vi "array of vectors -- algebra.vi"(4 "Array in":dbl[](array[numeric])=[0.1, 0.25, 0.5, 0.75, 1.25, 1.5], 6 "number":dbl=1.0, 7 "?":T2=enum."random", 8 "vec IN":cluster{"center x":dbl, "center Y":dbl}, 9 "Matrix":T1, 10 "y IN":dbl[](array[numeric])=[0.0, 0.0, 0.0, 0.0, 0.0, 0.0, 0.0, 0.0, 0.0, 0.0, 0.0, 0.0, 0.0, 0.0, 0.0, 0.0, 0.0, 0.0, 0.0, 0.0], 11 "x IN":dbl[](array[numeric])=[0.0, 0.0, 0.0, 0.0, 0.0, 0.0, 0.0, 0.0, 0.0, 0.0, 0.0, 0.0, 0.0, 0.0, 0.0, 0.0, 0.0, 0.0, 0.0, 0.0]) -> (0 "z out":dbl[](array[numeric]), 2 "y IOUT":dbl[](array[numeric])=[-0.10773170361060114, 0.457772952697413, -0.009555100977947983, -0.48804447463777656, -0.09984232901729184, 0.13119560893774174, -0.22283442709873946, 0.3059520406815761, -0.2724761090008474, 0.4459726318517574, 0.374683420003999, 0.15733456556750114, -0.2681733941926512, -0.18835513867488007, 0.201519355363871, -0.42899488425478816, 0.017153200329568463, -0.07357806321342775, -0.03965505008312653, -0.24040362888086708, 0.034052108855892715, 0.31924689447313703, -0.10598568269389563, -0.4403683770100004, -0.39067866845839583, -0.07628563470535954, 0.4798388214319522, 0.11632430011978867, 0.028320122257029068, -0.3713197715201815, 0.3687635262719211, -0.1672236935026572, -0.17019816064120863, 0.2670856862236137, -0.018456225948212834, -0.3697432881980798, 0.45329130138320917, 0.291174819494997, -0.4775794640153177, 0.20278732148372658, 0.00010603725885349746, -0.2782732301335482, -0.3370559874481738, -0.03489202794563595, 0.0441236466978302, 0.014425835304824552, 0.25050858523876185, 0.04621463682703997, 0.3475519129062037, 0.20029679806376333], 3 "x  OUT":dbl[](array[numeric])=[0.40090360765964794, 0.40170449063806646, 0.3719833615168324, -0.41942074860305834, 0.23408694456181145, 0.2004301402449875, -0.27413414162219407, 0.3227096166685155, -0.13636471969040254, -0.3615712316380595, -0.30837390549735244, -0.4972725670503759, 0.4538715795393323, -0.28219588600377743, -0.015344431033755601, -0.03162125419338757, 0.10462141481001197, -0.2184998697199254, -0.22600023642322253, -0.4336430625371366, -0.35474597926419627, -0.17008105009388963, 0.11680613183230104, -0.3147381858650824, 0.01810260701745814, 0.08118463453483504, 0.13197188439702667, -0.21774239766248127, -0.11943352032855747, 0.2300723285374393, 0.2763664885251238, -0.007778949200884622, 0.43387299574285265, 0.4591137756966033, 0.2612719864618036, -0.012468509690670038, -0.45450783010510687, -0.016721282298933993, -0.2893390780903706, 0.06254002811272952, 0.40529670225894754, -0.18315282359791607, 0.24745070704533223, 0.19736719755441556, -0.06565361009683168, 0.3076490949601618, -0.027569391016634803, -0.41363424870437493, 0.028513782340929383, 0.3932763712837244])   [LabVIEW 2021]
uses:
  array of vectors -- algebra.ctl
  <vilib>/Analysis/Matrix/Datatypes/RealMatrix.ctl
  generate linear region.vi
  <vilib>/Analysis/Matrix/NI_Matrix.lvlib
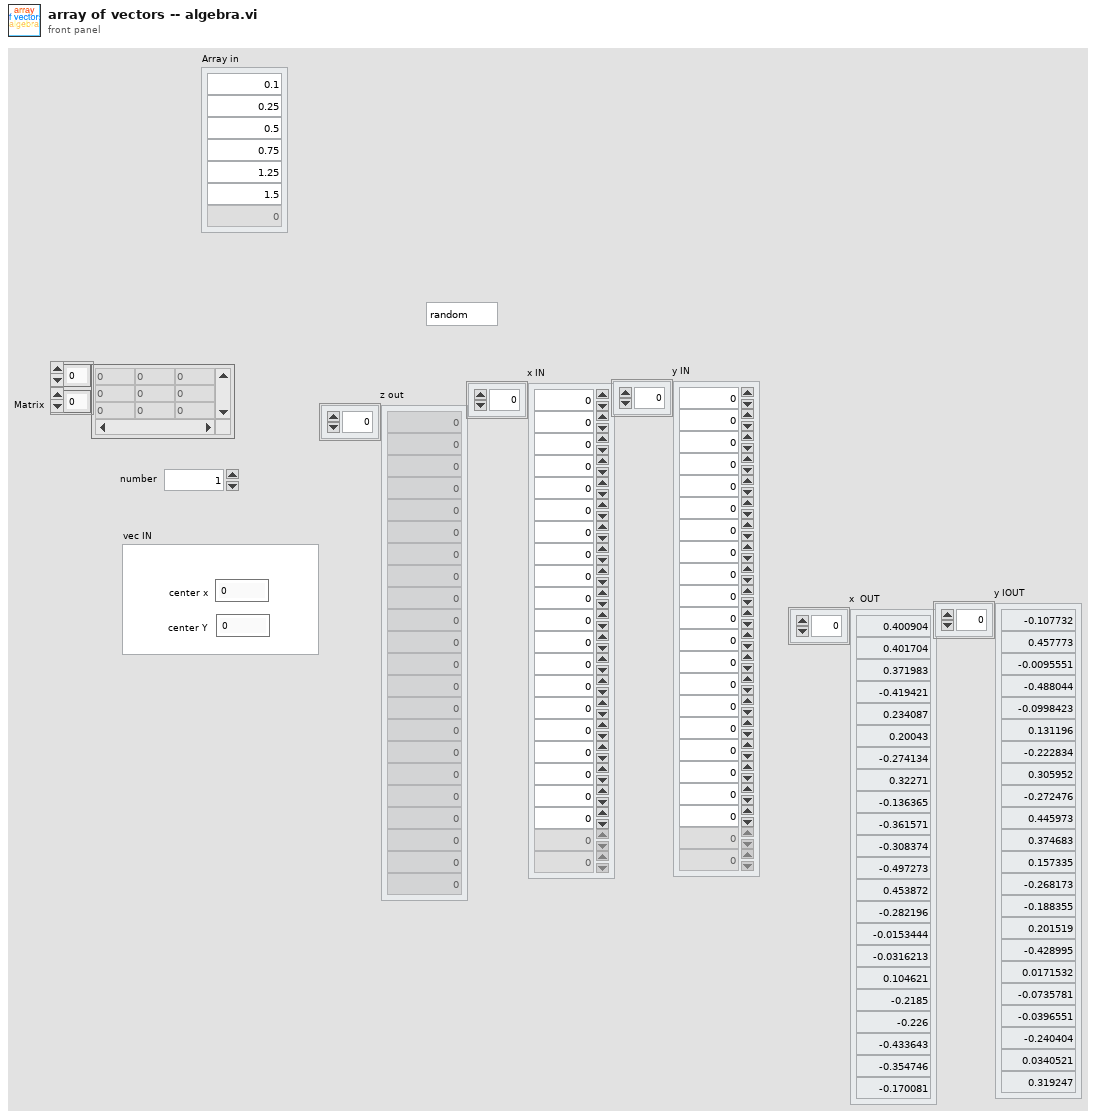
[diagram p1: front panel]
types:
  T1 = typedef "NI_Matrix.lvlib/RealMatrix.ctl" = dbl[][]
  T2 = typedef "array of vectors -- algebra.ctl" = enum16{"shift", "rotate", "scale", "multiply", "expectation", "random", "circles", ""}
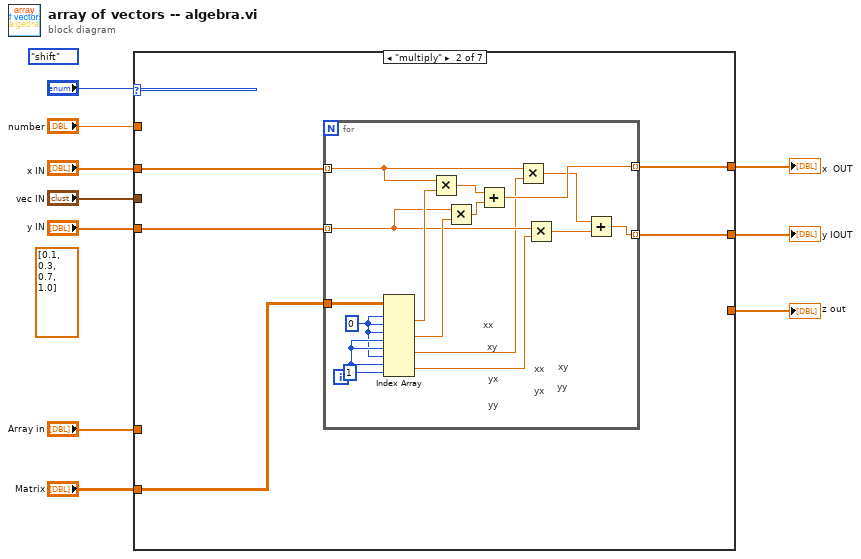
[diagram p0: block diagram]
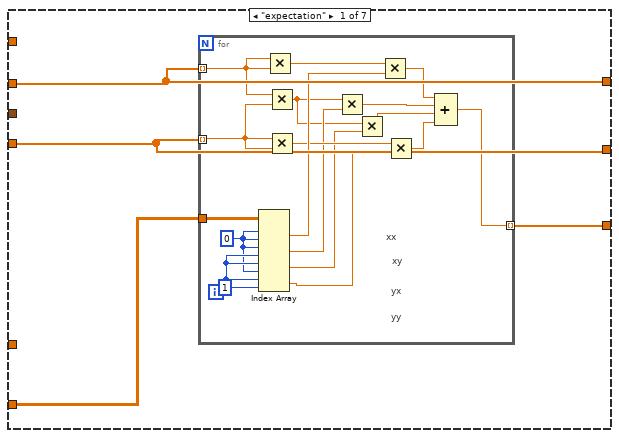
[diagram p2: hidden frame]
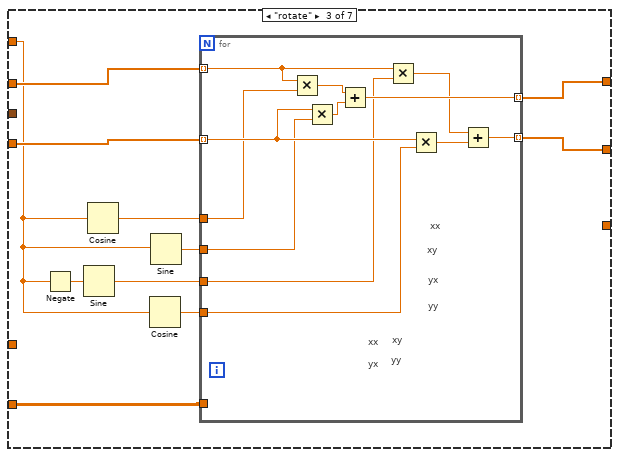
[diagram p3: hidden frame]
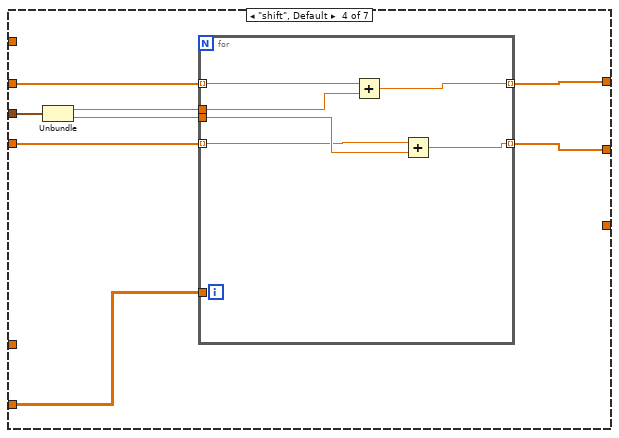
[diagram p4: hidden frame]
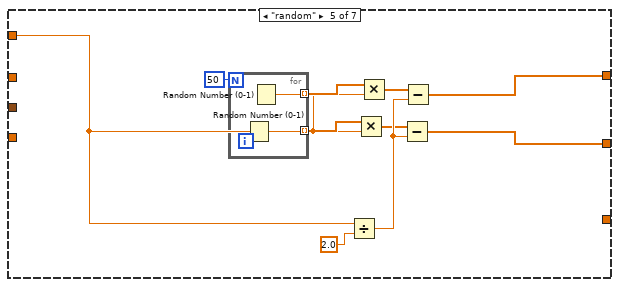
[diagram p5: hidden frame]
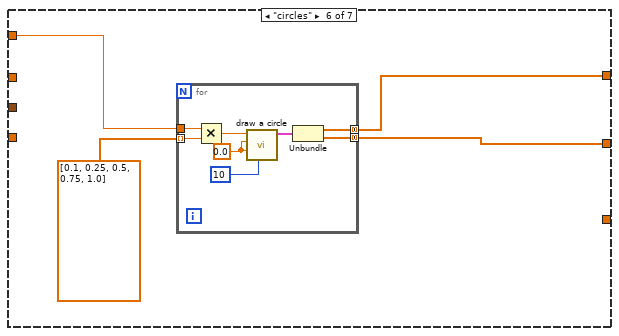
[diagram p6: hidden frame]
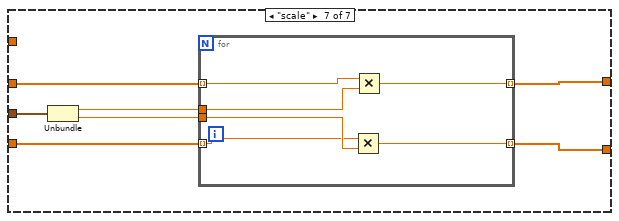
[diagram p7: hidden frame]
diagram:
  (unwired) dbl[] [0.1, 0.3, 0.7, 1.0]
  (unwired) array_of_vectors_--_algebra."shift"
  n1 = case shown="\"multiply\"" "?" {
    tunnel: "x IN" -> [w12 w36 w62 w82 _ _ w119]
    tunnel: "Matrix" -> [w14 w35 w61 w81 _ _ _]
    tunnel: [w13 _ _ _ _ _ _] -> w8
    tunnel: "y IN" -> [w11 w34 w60 w80 _ _ w118]
    tunnel: [w12 w33 w59 w79 w90 w103 w117] -> w5
    tunnel: [w11 w32 w58 w78 w89 w102 w116] -> w4
    tunnel: "number" -> [_ _ w53 _ w91 w104 _]
    tunnel: "vec IN" -> [_ _ _ w77 _ _ w113]
    tunnel: "Array in" -> [_ _ _ _ _ _ _]
    frame "expectation" {
      n2 = for {
        tunnel: w12 -> [w30] mode=indexing
        tunnel: w11 -> [w29] mode=indexing
        tunnel: w14 -> [w31]
        tunnel: [w23] -> w13 mode=indexing
        w22 = 1 ("index (row)")
        w21 = 0 ("index (row)")
        # "yy"
        # "yx"
        # "xy"
        # "xx"
        n3 = Index Array(array=w31, index (row) #1=w21, index (col) #1=w21, index (row) #2=w21, index (col) #2=w22, index (row) #3=w22, index (col) #3=w21, index (row) #4=w22, index (col) #4=w22) -> (element #1=w27:dbl, element #2=w25:dbl, element #3=w19:dbl, element #4=w18:dbl)
        n4 = Multiply(x=w30, y=w30) -> (x*y=w28:dbl)
        n5 = Multiply(x=w30, y=w29) -> (x*y=w20:dbl)
        n6 = Multiply(x=w29, y=w29) -> (x*y=w26:dbl)
        n7 = Multiply(x=w20, y=w25) -> (x*y=w15:dbl)
        n8 = Multiply(x=w20, y=w19) -> (x*y=w16:dbl)
        n9 = Multiply(x=w28, y=w27) -> (x*y=w24:dbl)
        n10 = Multiply ("Multiply.vi")(x=w26, y=w18) -> (x*y=w17:dbl)
        n11 = Compound Arithmetic op=ADD(w24, w15, w16, w17) -> (w23:dbl)
      }
    }
    frame "multiply" {
      n12 = for {
        tunnel: w36 -> [w40] mode=indexing
        tunnel: w34 -> [w39] mode=indexing
        tunnel: w35 -> [w51]
        tunnel: [w44] -> w33 mode=indexing
        tunnel: [w41] -> w32 mode=indexing
        w50 = 1 ("index (row)")
        w49 = 0 ("index (row)")
        # "yy"
        # "yx"
        # "xy"
        # "xx"
        # "yy"
        # "yx"
        # "xy"
        # "xx"
        n13 = Index Array(array=w51, index (row) #1=w49, index (col) #1=w49, index (row) #2=w49, index (col) #2=w50, index (row) #3=w50, index (col) #3=w49, index (row) #4=w50, index (col) #4=w50) -> (element #1=w48:dbl, element #2=w47:dbl, element #3=w38:dbl, element #4=w37:dbl)
        n14 = Multiply(x=w40, y=w48) -> (x*y=w46:dbl)
        n15 = Multiply(x=w39, y=w47) -> (x*y=w45:dbl)
        n16 = Add(x=w46, y=w45) -> (x+y=w44:dbl)
        n17 = Multiply(x=w40, y=w38) -> (x*y=w43:dbl)
        n18 = Multiply(x=w39, y=w37) -> (x*y=w42:dbl)
        n19 = Add(x=w43, y=w42) -> (x+y=w41:dbl)
      }
    }
    frame "rotate" {
      n20 = Negate(x=w53) -> (-x=w52:dbl)
      n21 = Sine(x=w52) -> (sin(x)=w55:dbl)
      n22 = Cosine(x=w53) -> (cos(x)=w56:dbl)
      n23 = Cosine(x=w53) -> (cos(x)=w57:dbl)
      n24 = Sine(x=w53) -> (sin(x)=w54:dbl)
      n25 = for {
        tunnel: w62 -> [w68] mode=indexing
        tunnel: w60 -> [w67] mode=indexing
        tunnel: w61 -> [_]
        tunnel: [w72] -> w59 mode=indexing
        tunnel: [w69] -> w58 mode=indexing
        tunnel: w57 -> [w66]
        tunnel: w56 -> [w65]
        tunnel: w55 -> [w64]
        tunnel: w54 -> [w63]
        # "yy"
        # "yx"
        # "xy"
        # "xx"
        # "yy"
        # "yx"
        # "xy"
        # "xx"
        n26 = Multiply(x=w68, y=w65) -> (x*y=w74:dbl)
        n27 = Multiply(x=w67, y=w63) -> (x*y=w73:dbl)
        n28 = Add(x=w74, y=w73) -> (x+y=w72:dbl)
        n29 = Multiply(x=w68, y=w64) -> (x*y=w71:dbl)
        n30 = Multiply(x=w67, y=w66) -> (x*y=w70:dbl)
        n31 = Add(x=w71, y=w70) -> (x+y=w69:dbl)
      }
    }
    frame "shift", Default {
      n32 = Unbundle(w77) -> ("center x"=w76:dbl, "center Y"=w75:dbl)
      n33 = for {
        tunnel: w82 -> [w86] mode=indexing
        tunnel: w80 -> [w83] mode=indexing
        tunnel: w81 -> [_]
        tunnel: [w88] -> w79 mode=indexing
        tunnel: [w87] -> w78 mode=indexing
        tunnel: w76 -> [w85]
        tunnel: w75 -> [w84]
        n34 = Add(x=w86, y=w85) -> (x+y=w88:dbl)
        n35 = Add(x=w83, y=w84) -> (x+y=w87:dbl)
      }
    }
    frame "random" {
      n36 = for {
        N: 50 -> [_]
        tunnel: [w100] -> w95 mode=indexing
        tunnel: [w99] -> w94 mode=indexing
        n37 = Random Number (0-1)() -> (number: 0 to 1=w99:dbl)
        n38 = Random Number (0-1)() -> (number: 0 to 1=w100:dbl)
      }
      n39 = Divide(x=w91, y=2.0) -> (x/y=w98:dbl)
      n40 = Multiply(x=w94, y=w91) -> (x*y=w97:dbl[])
      n41 = Multiply(x=w95, y=w91) -> (x*y=w96:dbl[])
      n42 = Subtract(x=w97, y=w98) -> (x-y=w89:dbl[])
      n43 = Subtract(x=w96, y=w98) -> (x-y=w90:dbl[])
    }
    frame "circles" {
      n44 = for {
        tunnel: w104 -> [w107]
        tunnel: [w109] -> w103 mode=concatenating
        tunnel: [w108] -> w102 mode=concatenating
        tunnel: dbl[] [0.1, 0.25, 0.5, 0.75, 1.0] ("Array in") -> [w105] mode=indexing
        w110 = 0.0 ("center x")
        n45 = Multiply(x=w107, y=w105) -> (x*y=w106:dbl)
        n46 = call "draw a circle.vi"("number of points"=10, "center Y"=w110, "center x"=w110, "radius"=w106) -> ("output cluster"=w111:cluster{dbl[], dbl[]})  [unwired: 7 in]
        n47 = Unbundle(w111) -> (w109:dbl[], w108:dbl[])
      }
    }
    frame "scale" {
      n48 = Unbundle(w113) -> ("center x"=w115:dbl, "center Y"=w114:dbl)
      n49 = for {
        tunnel: w119 -> [w123] mode=indexing
        tunnel: w118 -> [w120] mode=indexing
        tunnel: [w125] -> w117 mode=indexing
        tunnel: [w124] -> w116 mode=indexing
        tunnel: w115 -> [w122]
        tunnel: w114 -> [w121]
        n50 = Multiply(x=w120, y=w121) -> (x*y=w124:dbl)
        n51 = Multiply(x=w123, y=w122) -> (x*y=w125:dbl)
      }
    }
  }
  "z out" <- w8
  "x  OUT" <- w5
  "y IOUT" <- w4
